vi "Global Mes Triger.vi"(8 "error in (no error)":errorcluster, 10 "R/S":bool, 11 "Var":T1) -> (0 "error out":errorcluster, 3 "Var out":T1)   [LabVIEW 2014]
uses:
  Type'def/Phone Var.ctl
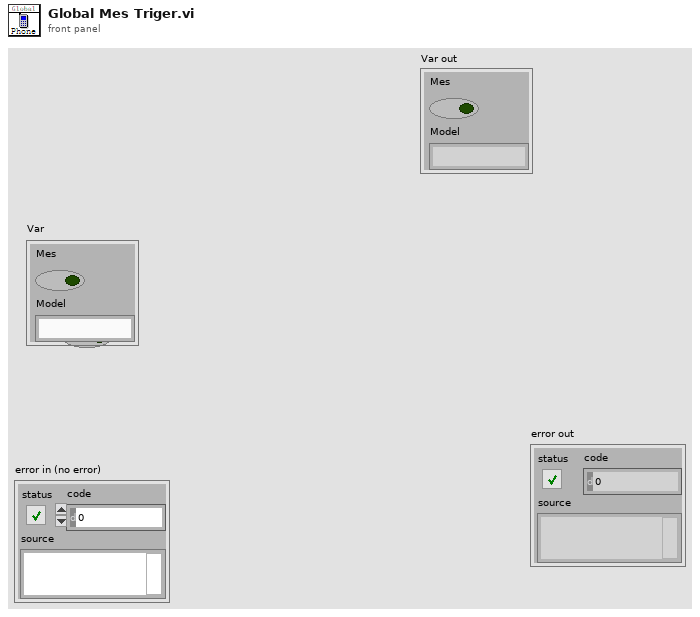
[diagram p1: front panel]
types:
  T1 = typedef "Phone Var.ctl" = cluster{"Mes":bool, "Model":string}
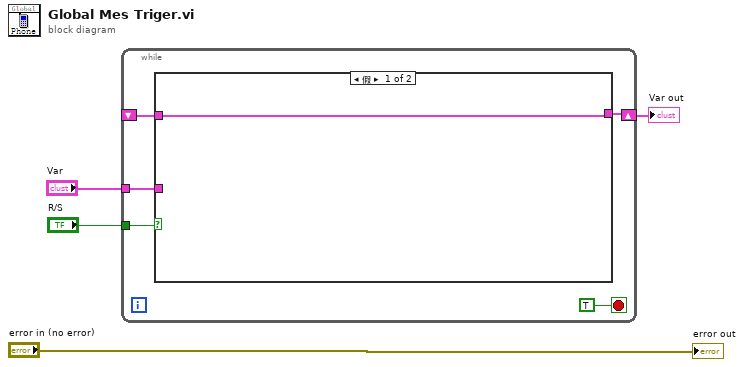
[diagram p0: block diagram]
diagram:
  n1 = while {
    tunnel: "R/S" -> [w8]
    tunnel: "Var" -> [w7]
    shift-right: [w6] -> w1
    shift-left: _ -> [w5]
    stop <- TRUE stop-if-true
    n2 = case shown="假" w8 {
      tunnel: w7 -> [_ w11]
      tunnel: [w10 w11] -> w6
      tunnel: w5 -> [w10 _]
      frame False {
      }
      frame True {
      }
    }
  }
  "Var out" <- w1
  "error out" <- "error in (no error)"
